vi "Process and Save Data.vi"(7 "step#":u32, 8 "error in":errorcluster, 10 "New Data Array":dbl[](array[numeric]) format="%#_12g", 11 "Scan Driver.lvclass in":refnum<class "Scan Driver.lvclass">) -> (0 "error out":errorcluster, 1 "primary graph data":dbl[](array[numeric]), 2 "polarization graph data":dbl[](array[numeric]), 3 "Scan Driver.lvclass out":refnum<class "Scan Driver.lvclass">)   [LabVIEW 2009, in "Scan Driver.lvclass"]
doc: "(Deprecated) Given a new data point, generate one or more auxilliary data points from a secondary source, e.g. a modulator Instrument or an internal computation algorithm. Immediately write all data points to a temporay backup file."
uses:
  Scan Driver.lvclass
  Scan Driver.lvclass/Scan Driver.ctl
  <vilib>/Utility/file.llb/Write To Spreadsheet File (DBL).vi
  File IO/File IO.lvclass
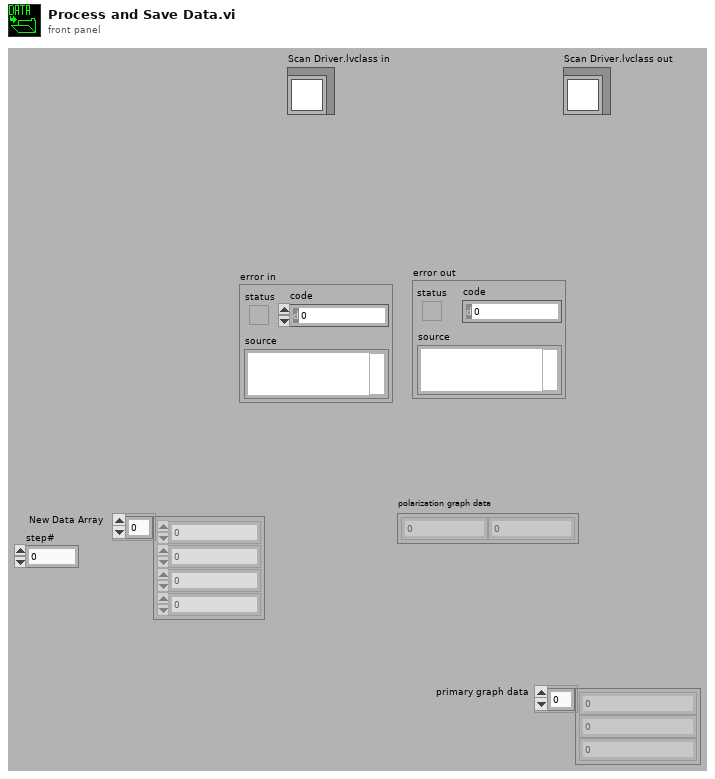
[diagram p1: front panel]
types:
  T1 = cluster{"Data Column Headings":string[], "Primary Plot Labels":string[], "Secondary Plot Labels":string[], "Tag":string, "Y-axis":string, "Total # Columns (incl. X-var)":dbl, "Index of first Secondary\nColumn (from 0)":dbl, "# Secondary Columns":dbl, "# Data Columns (deprecated)":dbl, "# Data Columns":dbl}
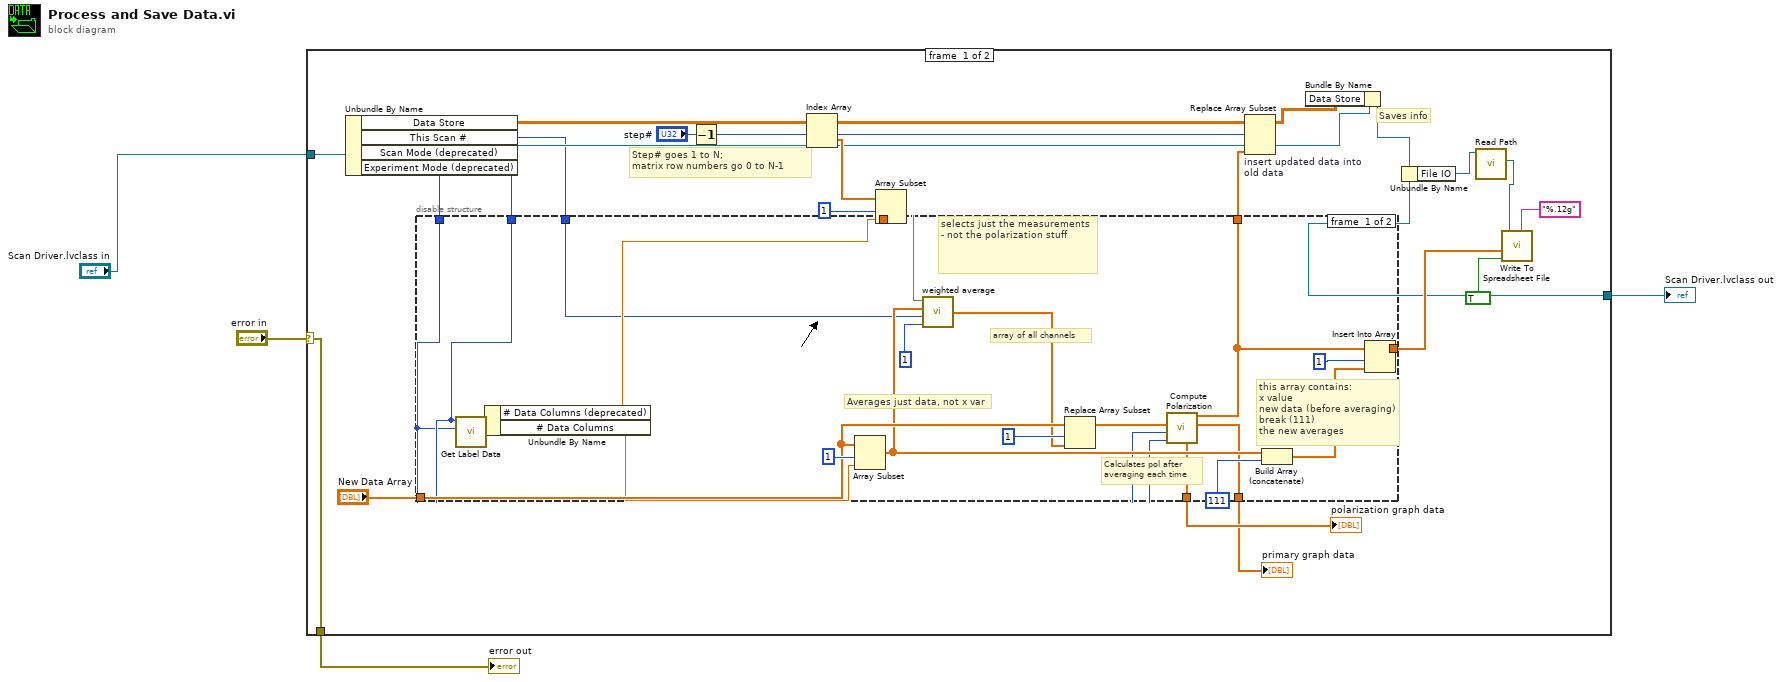
[diagram p0: block diagram]
diagram:
  n1 = case shown="No Error" "error in" {
    selector: "error in" -> [w15 w49]
    tunnel: [w15 w49] -> w3
    tunnel: "Scan Driver.lvclass in" -> [w14 w50]
    tunnel: [w8 w50] -> w1
    frame #0 {
      # "Step# goes 1 to N;\nmatrix row numbers go 0 to N-1"
      # "Saves info"
      n2 = Unbundle By Name(w14) -> ("Data Store"=w13:dbl[][], "This Scan #"=w9:u32, "Scan Mode (deprecated)"=w11:u8, "Experiment Mode (deprecated)"=w10:u8)
      n3 = Decrement(x="step#") -> (x-1=w5:u32)
      n4 = Index Array(array=w13, index (row)=w5) -> (element=w24:dbl[])  [unwired: 1 in]
      n5 = disable-structure shown="Enabled" {
        disable-tunnel: w24 -> [w45 _]
        disable-tunnel: "New Data Array" -> [w41 w48]
        disable-tunnel: [w38 w48] -> w20
        disable-tunnel: [w33 w48] -> w19
        disable-tunnel: [w32 w48] -> w18
        disable-tunnel: [w31 w48] -> w17
        disable-tunnel: w11 -> [w27 _]
        disable-tunnel: w10 -> [w26 _]
        disable-tunnel: w9 -> [w25 _]
        frame #0 {
          # "this array contains:\nx value\nnew data (before averaging)\nbreak (111)\nthe new averages"
          # "selects just the measurements - not the polarization stuff"
          # "array of all channels"
          # "Calculates pol after\naveraging each time"
          # "Averages just data, not x var"
          n6 = call "Get Label Data.vi"("expmode"=w26, "scanmode"=w27) -> ("data"=w28:T1)  [unwired: 9 out]
          n7 = Unbundle By Name(w28) -> ("# Data Columns (deprecated)"=w29:dbl, "# Data Columns"=w30:dbl)
          n8 = Array Subset(array=w41, index=1, length=w30) -> (w36:dbl[])
          n9 = Array Subset(array=w45, index=1, length=w29) -> (w46:dbl[])
          n10 = call "weighted average.vi"("WeightB"=1, "WeightA"=w25, "NumberB"=w36, "NumberA"=w46) -> ("Avg"=w40:dbl[])
          n11 = Replace Array Subset(array=w41, new element=w40, index=1) -> (w39:dbl[])
          n12 = call "Compute Polarization.vi"("expmode"=w26, "scanmode"=w27, "arraydata"=w39) -> ("plotdata"=w31:dbl[], "savedata"=w38:dbl[], "poldisplay"=w32:dbl[])  [unwired: 6 out]
          n13 = Build Array (concatenate)(w36, 111) -> (w35:dbl[])
          n14 = Insert Into Array(array=w38, index=1, new element=w35) -> (w33:dbl[])
        }
        frame #1 {
          # "XXX 02-11-2010 SB\nPolarization doesn't work\n(deps on ScanMode/ExpMode)\nBypass for now and send all\ndata to both graphs and outfile"
        }
      }
      "primary graph data" <- w17
      "polarization graph data" <- w18
      n15 = Replace Array Subset "insert updated data into old data"(array=w13, new element=w20, index (row)=w5) -> (w12:dbl[][])  [unwired: 1 in]
      n16 = Bundle By Name(cluster=w14, "Data Store"=w12) -> (w8:refnum<class "Scan Driver.lvclass">)
      n17 = Unbundle By Name(w8) -> ("File IO"=w7:refnum<class "File IO.lvclass">)
      n18 = call-dynamic "Read Path.vi"("File IO.lvclass in"=w7) -> ("Temporary Path"=w6:path)  [unwired: 1 in, 9 out]
      n19 = call-poly <vilib>:"Write To Spreadsheet File.vi"("format (%.3f)"="%.12g", "append to file? (new file:F)"=TRUE, "1D data"=w19, "file path (dialog if empty)"=w6) -> ()  [unwired: 2 in, 3 out]
    }
    frame #1 {
    }
  }
  "Scan Driver.lvclass out" <- w1
  "error out" <- w3
